vi "Tickcount.vi"() -> ()   [LabVIEW 2019]
panel:
  in  "stop":bool
  out "millisecond timer value":u32
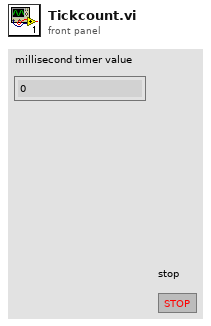
[diagram p1: front panel]
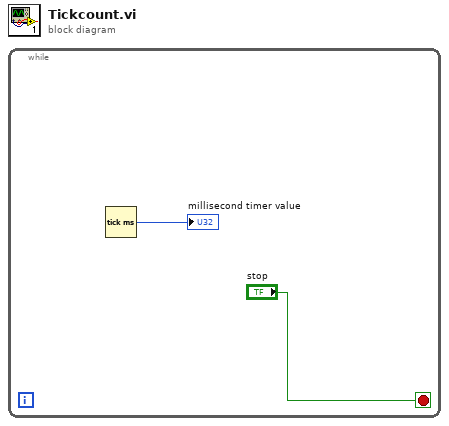
[diagram p0: block diagram]
diagram:
  n1 = while {
    stop <- "stop" stop-if-true
    n2 = Tick Count (ms)() -> (millisecond timer value=→"millisecond timer value":u32)
  }
